vi "Write Panel.vi"(8 "error in (no error)":errorcluster, 10 "Panel.lvlib:Panel.lvclass":refnum<class "Panel.lvclass">, 11 "Panel Actor Form Config in":refnum<class "Panel Actor Form Config.lvclass">) -> (0 "error out":errorcluster, 3 "Panel Actor Form Config out":refnum<class "Panel Actor Form Config.lvclass">)   [LabVIEW 2020, in "Panel Actor Form Config.lvclass"]
uses:
  Panel Actor Form Config.lvclass
  <vilib>/MGI/Panel Manager/Panel/Panel/Panel.lvclass
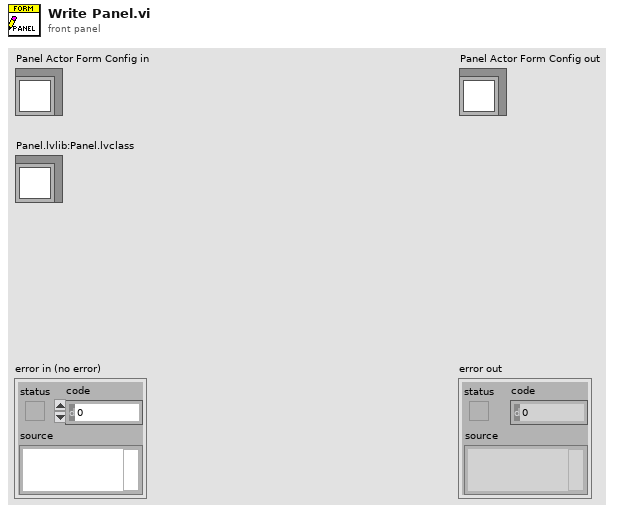
[diagram p1: front panel]
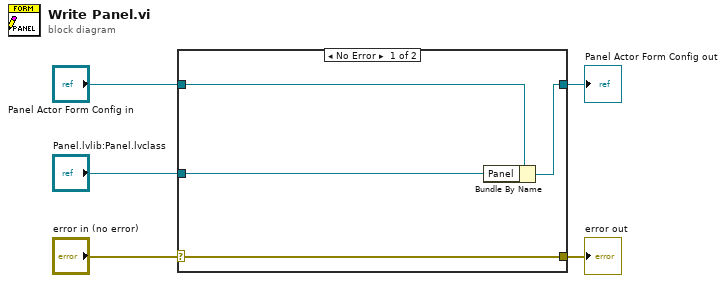
[diagram p0: block diagram]
diagram:
  n1 = case shown="No Error" "error in (no error)" {
    selector: "error in (no error)" -> [w9 w10]
    tunnel: [w9 w10] -> w4
    tunnel: [w7 w11] -> w2
    tunnel: "Panel Actor Form Config in" -> [w8 w11]
    tunnel: "Panel.lvlib:Panel.lvclass" -> [w6 _]
    frame No Error {
      n2 = Bundle By Name(cluster=w8, "Panel"=w6) -> (w7:refnum<class "Panel Actor Form Config.lvclass">)
    }
    frame Error {
    }
  }
  "error out" <- w4
  "Panel Actor Form Config out" <- w2
